vi "Write DAC.vi"(8 "error in (no error)":errorcluster, 9 "Analog Output V1":u16, 10 "Analog Output VO":u16, 11 "RGB in":refnum<class "An Out I2C.lvclass">) -> (0 "error out":errorcluster, 3 "RGB out":refnum<class "An Out I2C.lvclass">)   [LabVIEW 2020, in "CTI-Peripheral.lvlib" / "An Out I2C.lvclass"]
uses:
  An Out I2C.lvclass
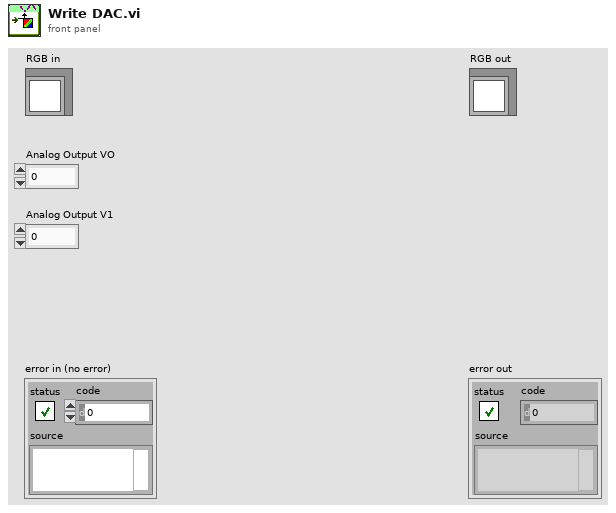
[diagram p1: front panel]
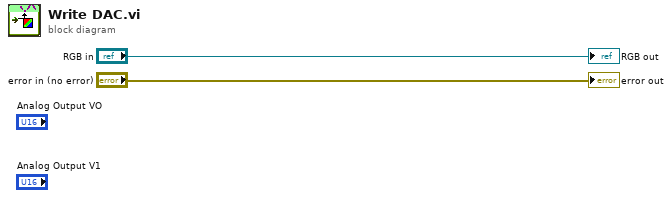
[diagram p0: block diagram]
diagram:
  "error out" <- "error in (no error)"
  "RGB out" <- "RGB in"
